vi "ItemsOfType.vi"(7 "LabVIEW Object Type":refnum<class>, 8 "error in (no error)":errorcluster, 11 "Collection in":refnum<class "CollectionByValue.lvclass">) -> (0 "error out":errorcluster, 1 "found":bool, 2 "LabVIEW Objects":refnum<class>[](array[class]), 3 "Collection out":refnum<class "CollectionByValue.lvclass">)   [LabVIEW 2021, in "Collection.lvlib" / "CollectionByValue.lvclass"]
uses:
  CollectionByValue.lvclass
  CollectionByValue.lvclass/CollectionByValue.ctl
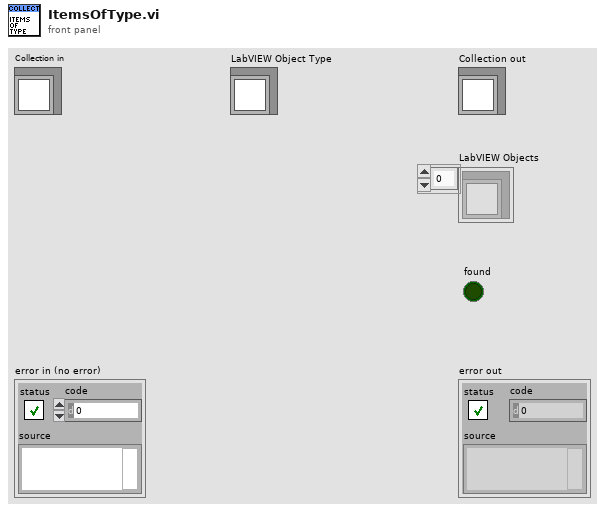
[diagram p1: front panel]
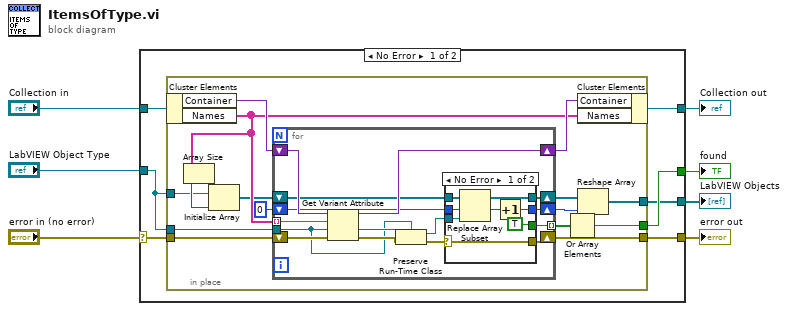
[diagram p0: block diagram]
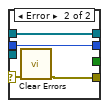
[diagram p2: hidden frame]
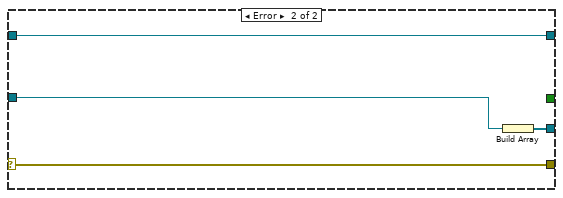
[diagram p3: hidden frame]
diagram:
  n1 = case shown="No Error" "error in (no error)" {
    selector: "error in (no error)" -> [w12 w59]
    tunnel: [w11 w59] -> w6
    tunnel: [w13 w58] -> w4
    tunnel: "Collection in" -> [w14 w58]
    tunnel: "LabVIEW Object Type" -> [w9 w57]
    tunnel: [w10 _] -> w2
    tunnel: [w8 w56] -> w1
    frame No Error {
      n2 = in-place {
        in-place-border: w12 -> [w29]
        in-place-border: w9 -> [w25]
        in-place-border: [w26] -> w11
        in-place-border: [w15] -> w10
        in-place-border: w9 -> [w22]
        in-place-border: [w18] -> w8
        n3 = in-place-cluster #1(w14) -> ("Container"=w28:variant, "Names"=w23:string[])
        n4 = Array Size(array=w23) -> (size(s)=w24:i32)
        n5 = Initialize Array(w22, w24) -> (w21:refnum<class>[])
        n6 = for {
          tunnel: w23 -> [w43] mode=indexing
          tunnel: w25 -> [w33]
          shift-right: [w31] -> w26
          shift-left: w29 -> [w44]
          shift-right: [w41] -> w27
          shift-left: w28 -> [w42]
          shift-right: [w36] -> w19
          shift-left: w21 -> [w38]
          shift-right: [w32] -> w17
          shift-left: 0 -> [w37]
          tunnel: [w30] -> w16 mode=indexing
          n7 = Get Variant Attribute(Variant=w42, name=w43, default value (empty Variant)=w33, error in=w44) -> (duplicate Variant=w41:variant, value=w34:refnum<class>, error out=w35:errorcluster)  [unwired: 1 out]
          n8 = Preserve Run-Time Class(object in=w34, error in=w35, 2:w33) -> (object out=w39:refnum<class>, error out=w40:errorcluster)
          n9 = case shown="No Error" w40 {
            selector: w40 -> [w48 w53]
            tunnel: w39 -> [w49 _]
            tunnel: w38 -> [w51 w55]
            tunnel: w37 -> [w47 w54]
            tunnel: [w50 w55] -> w36
            tunnel: [w46 w54] -> w32
            tunnel: [w48 w52] -> w31
            tunnel: [TRUE _] -> w30
            frame No Error {
              n10 = Replace Array Subset(array=w51, new element=w49, index=w47) -> (w50:refnum<class>[])
              n11 = Increment(x=w47) -> (x+1=w46:i32)
            }
            frame Error {
              n12 = call <vilib>:"Clear Errors.vi"("error in (no error)"=w53) -> ("error out"=w52:errorcluster)  [unwired: 5 in, 1 out]
            }
          }
        }
        n13 = Or Array Elements(Boolean array=w16) -> (logical OR=w15:bool)
        n14 = in-place-cluster #1("Container"=w27, "Names"=w23) -> (w13:refnum<class "CollectionByValue.lvclass">)
        n15 = Reshape Array(w19, w17) -> (w18:refnum<class>[])
      }
    }
    frame Error {
      n16 = Build Array(w57) -> (w56:refnum<class>[])
    }
  }
  "error out" <- w6
  "Collection out" <- w4
  "LabVIEW Objects" <- w1
  "found" <- w2
